vi "RTS TCP Real Time.vi"(0 "Chamber 1 Socket":string[][](array[string]), 3 "All Data in":dbl[][](array[numeric]), 5 "Chamber 2 Socket":string[][](array[string]), 9 "Chamber 3 Socket":string[][](array[string]), 11 "error in (no error)":errorcluster, 12 "Chamber 4 Socket":string[][](array[string]), 14 "Tree Selection":T1) -> (1 "Full Item Names":string[](array[string]), 4 "Chamber Data":string[][](array[string]), 6 "All Data out":dbl[][](array[numeric]), 8 "Custom Titles":string[](array[string]), 10 "Listbox Data":string[][](array[string]), 13 "Point File Name":string, 15 "error out":errorcluster)   [LabVIEW 2020]
uses:
  Type Definitions/RTS Room Selector.ctl
  Type Definitions/RTS TDMS Data.ctl
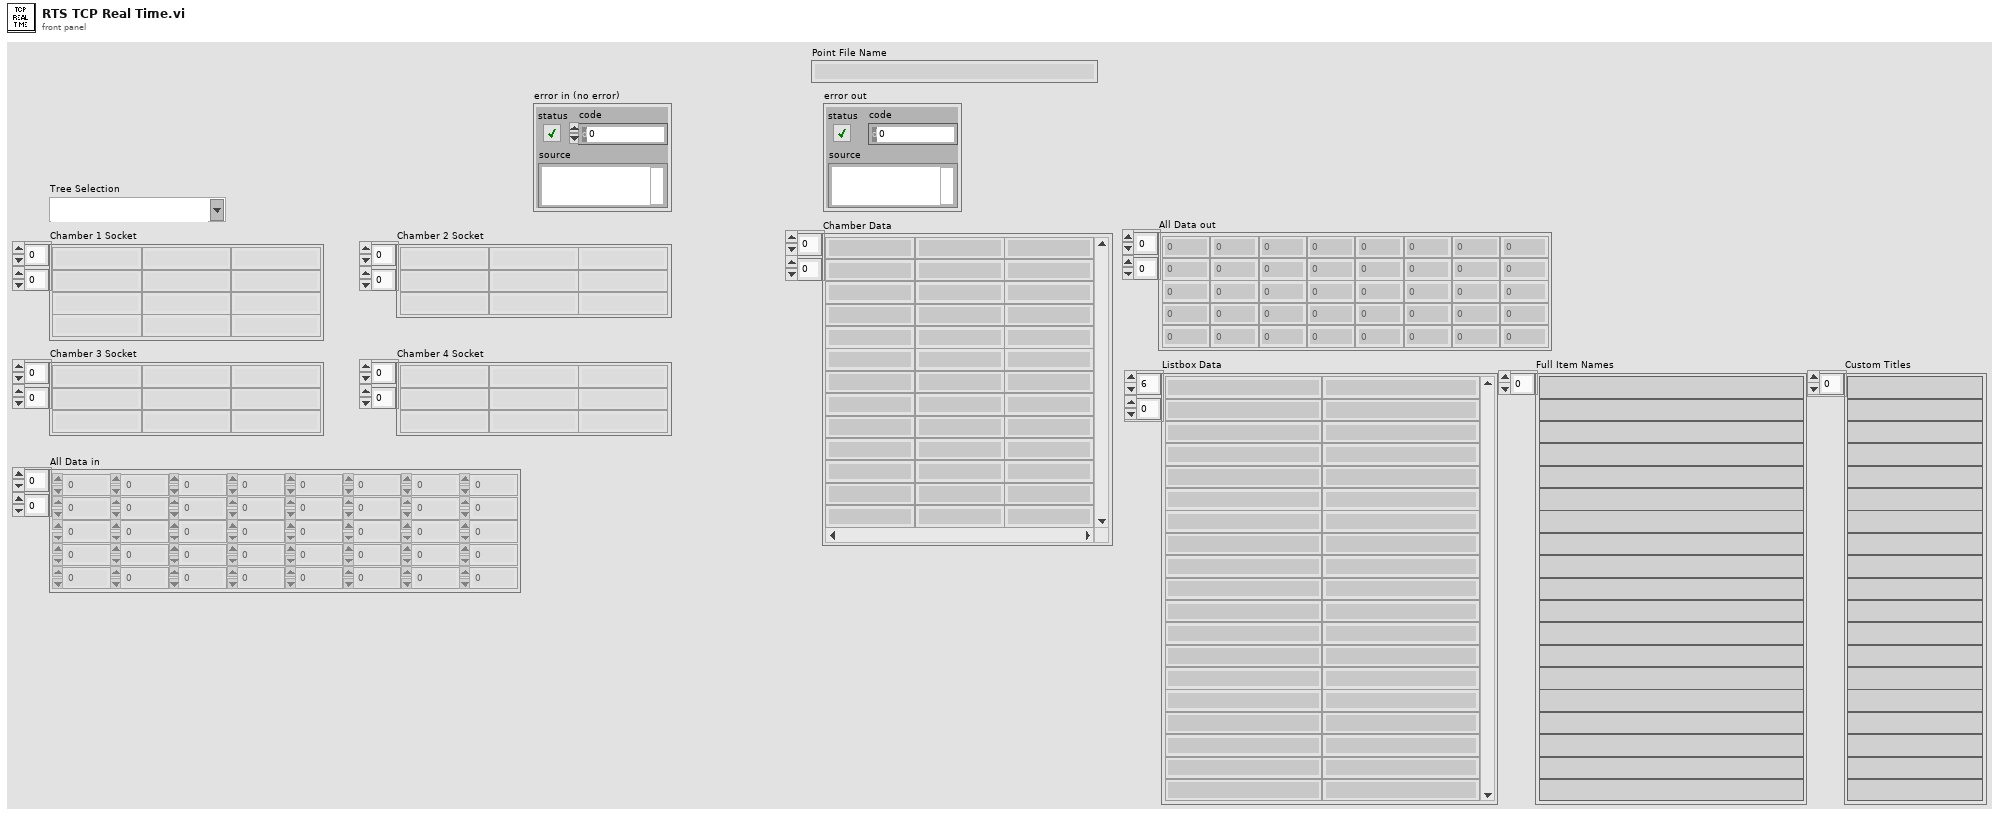
[diagram p1: front panel]
types:
  T1 = typedef "RTS Room Selector.ctl" = string
  T2 = typedef "RTS TDMS Data.ctl" = cluster{"Station 1":dbl[][], "Station 2":dbl[][], "Station 3":dbl[][], "Station 4":dbl[][], "Station 5":dbl[][], "Station 6":dbl[][], "Station 7":dbl[][], "Station 8":dbl[][]}
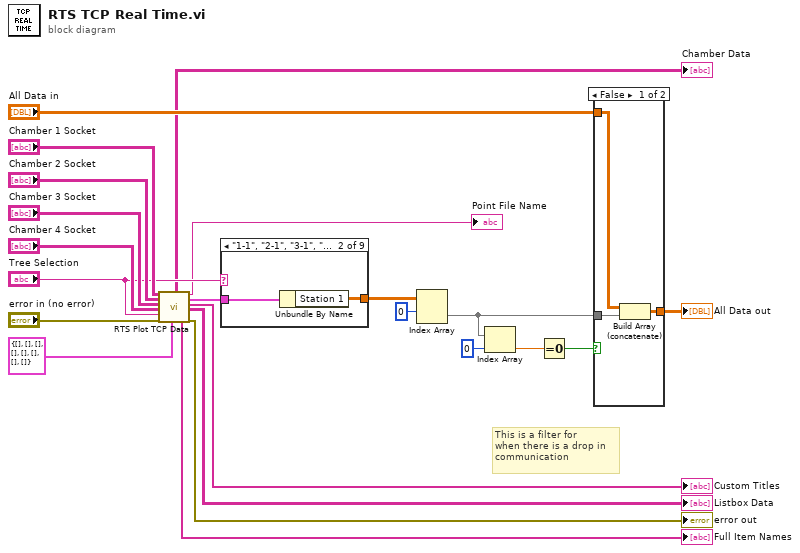
[diagram p0: block diagram]
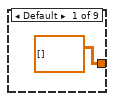
[diagram p3: hidden frame]
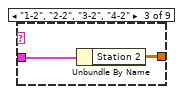
[diagram p4: hidden frame]
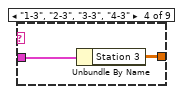
[diagram p5: hidden frame]
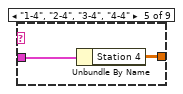
[diagram p6: hidden frame]
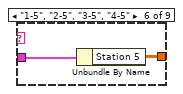
[diagram p7: hidden frame]
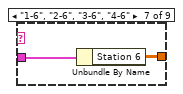
[diagram p8: hidden frame]
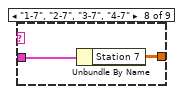
[diagram p9: hidden frame]
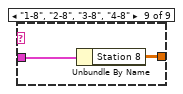
[diagram p10: hidden frame]
diagram:
  # "This is a filter for\nwhen there is a drop in \ncommunication"
  n1 = call "RTS Plot TCP Data.vi"("Chamber 1 Socket"="Chamber 1 Socket", "Chamber 2 Socket"="Chamber 2 Socket", "Chamber 3 Socket"="Chamber 3 Socket", "Chamber 4 Socket"="Chamber 4 Socket", "Tree Selection in"="Tree Selection", "Error In"="error in (no error)", "CSV Data in"=T2 {"Station 1"=[], "Station 2"=[], "Station 3"=[], "Station 4"=[], "Station 5"=[], "Station 6"=[], "Station 7"=[], "Station 8"=[]} ("CSV Data")) -> ("Chamber Data"=→"Chamber Data":string[][], "Full Item Names"=→"Full Item Names":string[], "Point File Name"=→"Point File Name":string, "CSV Data out"=w13:T2, "Custom Titles"=→"Custom Titles":string[], "Listbox Data"=→"Listbox Data":string[][], "Error Out"=→"error out":errorcluster)  [unwired: 5 in, 1 out]
  n2 = case shown="\"1-1\", \"2-1\", \"3-1\", \"4-1\"" "Tree Selection" {
    tunnel: [dbl[][] [] w25 w27 w29 w31 w33 w35 w37 w39] -> w7
    tunnel: w13 -> [_ w24 w26 w28 w30 w32 w34 w36 w38]
    frame Default {
    }
    frame "1-1", "2-1", "3-1", "4-1" {
      n3 = Unbundle By Name(w24) -> ("Station 1"=w25:dbl[][])
    }
    frame "1-2", "2-2", "3-2", "4-2" {
      n4 = Unbundle By Name(w26) -> ("Station 2"=w27:dbl[][])
    }
    frame "1-3", "2-3", "3-3", "4-3" {
      n5 = Unbundle By Name(w28) -> ("Station 3"=w29:dbl[][])
    }
    frame "1-4", "2-4", "3-4", "4-4" {
      n6 = Unbundle By Name(w30) -> ("Station 4"=w31:dbl[][])
    }
    frame "1-5", "2-5", "3-5", "4-5" {
      n7 = Unbundle By Name(w32) -> ("Station 5"=w33:dbl[][])
    }
    frame "1-6", "2-6", "3-6", "4-6" {
      n8 = Unbundle By Name(w34) -> ("Station 6"=w35:dbl[][])
    }
    frame "1-7", "2-7", "3-7", "4-7" {
      n9 = Unbundle By Name(w36) -> ("Station 7"=w37:dbl[][])
    }
    frame "1-8", "2-8", "3-8", "4-8" {
      n10 = Unbundle By Name(w38) -> ("Station 8"=w39:dbl[][])
    }
  }
  n11 = Index Array(array=w7, index (row)=0) -> (element=w18:dbl[])  [unwired: 1 in]
  n12 = Index Array(array=w18, index=0) -> (element=w20:dbl)
  n13 = Equal To 0?(x=w20) -> (x = 0?=w21:bool)
  n14 = case shown="False" w21 {
    tunnel: "All Data in" -> [w42 w43]
    tunnel: [w41 w43] -> w12
    tunnel: w18 -> [w40 _]
    frame False {
      n15 = Build Array (concatenate)(w42, w40) -> (w41:dbl[][])
    }
    frame True {
    }
  }
  "All Data out" <- w12
